vi "Get Session Information.vi"(8 "error in (no error)":errorcluster, 11 "reserve sessions response":T4) -> (0 "error out":errorcluster, 3 "session information":T1)   [LabVIEW 2020, in "Keysight 34401A DMM Measurement.lvlib"]
uses:
  Keysight 34401A DMM Measurement.lvlib
  <vilib>/MeasurementLink/MeasurementLink Session Management Client/RPC Messages/ni_measurementlink_sessionmanagement_v1_ReserveSessionsResponse.ctl
  <vilib>/MeasurementLink/MeasurementLink Session Management Client/RPC Messages/ni_measurementlink_sessionmanagement_v1_SessionInformation.ctl
  <vilib>/MeasurementLink/MeasurementLink Session Management Client/RPC Messages/nidevice_grpc_Session.ctl
  <vilib>/MeasurementLink/MeasurementLink Session Management Client/RPC Messages/ni_measurementlink_sessionmanagement_v1_ChannelMapping.ctl
  <vilib>/MeasurementLink/MeasurementLink Session Management Client/MeasurementLink Session Management Client.lvlib
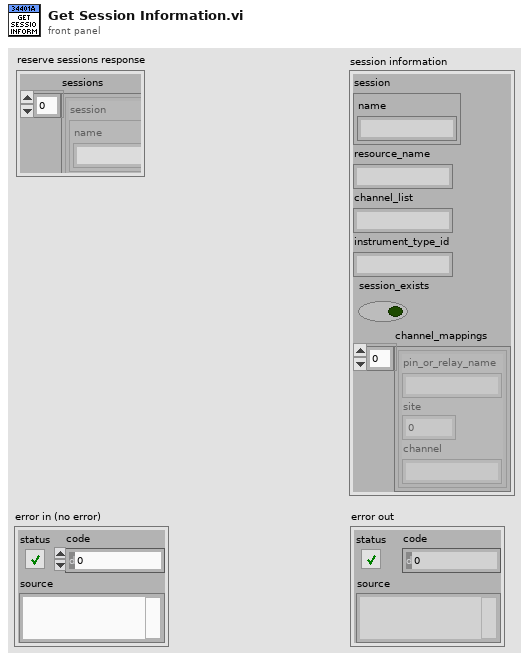
[diagram p1: front panel]
types:
  T1 = typedef "MeasurementLink Session Management Client.lvlib/ni_measurementlink_sessionmanagement_v1_SessionInformation.ctl" = cluster{"session":T2, "resource_name":string, "channel_list":string, "instrument_type_id":string, "session_exists":bool, "channel_mappings":T3[]}
  T2 = typedef "MeasurementLink Session Management Client.lvlib/nidevice_grpc_Session.ctl" = cluster{"name":string}
  T3 = typedef "MeasurementLink Session Management Client.lvlib/ni_measurementlink_sessionmanagement_v1_ChannelMapping.ctl" = cluster{"pin_or_relay_name":string, "site":i32, "channel":string}
  T4 = typedef "MeasurementLink Session Management Client.lvlib/ni_measurementlink_sessionmanagement_v1_ReserveSessionsResponse.ctl" = cluster{"sessions":T1[]}
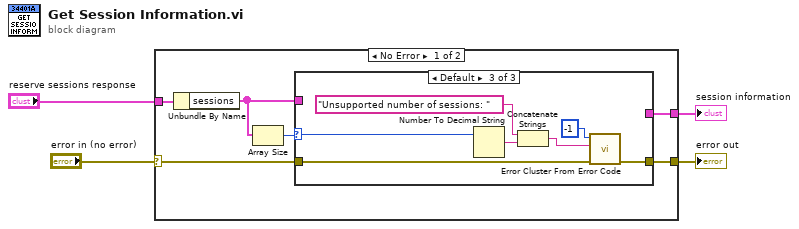
[diagram p0: block diagram]
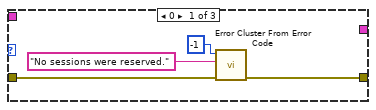
[diagram p2: hidden frame]
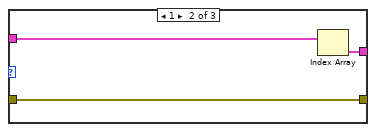
[diagram p3: hidden frame]
diagram:
  n1 = case shown="No Error" "error in (no error)" {
    selector: "error in (no error)" -> [w8 w25]
    tunnel: "reserve sessions response" -> [w10 _]
    tunnel: [w7 w25] -> w2
    tunnel: [w5 _] -> w1
    frame No Error {
      n2 = Unbundle By Name(w10) -> ("sessions"=w6:T1[])
      n3 = Array Size(array=w6) -> (size(s)=w9:i32)
      n4 = case shown="Default" w9 {
        selector: w9 -> [_ _ w19]
        tunnel: w8 -> [w14 w15 w24]
        tunnel: [w11 w15 w22] -> w7
        tunnel: w6 -> [_ w17 _]
        tunnel: [_ w16 _] -> w5
        frame 0 {
          n5 = call <vilib>:"Error Cluster From Error Code.vi"("error in (no error)"=w14, "error message (\"\")"="No sessions were reserved." ("error message (\"\")"), "error code (0)"=-1) -> ("error out"=w11:errorcluster)  [unwired: 6 in]
        }
        frame 1 {
          n6 = Index Array(array=w17) -> (element=w16:T1)  [unwired: 1 in]
        }
        frame Default {
          n7 = Number To Decimal String(number=w19) -> (decimal integer string=w20:string)  [unwired: 1 in]
          n8 = Concatenate Strings("Unsupported number of sessions: " ("error message (\"\")"), w20) -> (w18:string)
          n9 = call <vilib>:"Error Cluster From Error Code.vi"("error in (no error)"=w24, "error message (\"\")"=w18, "error code (0)"=-1) -> ("error out"=w22:errorcluster)  [unwired: 6 in]
        }
      }
    }
    frame Error {
    }
  }
  "error out" <- w2
  "session information" <- w1
